vi "Recipe Label Changed-Event.vi"(8 "error in (no error)":errorcluster, 10 "New Label":string, 11 "Recipe Window in":refnum<class "Recipe Window.lvclass">) -> (0 "error out":errorcluster, 3 "Recipe Window out":refnum<class "Recipe Window.lvclass">)   [LabVIEW 2021, in "Recipe.lvlib" / "Recipe Window.lvclass"]
uses:
  Recipe Window.lvclass
  C:/Program Files (x86)/National Instruments/LabVIEW 2021/vi.lib/MGI/Monitored Actor/Monitored Actor/Monitored Actor/Monitored Actor.lvclass
  C:/Program Files (x86)/National Instruments/LabVIEW 2021/vi.lib/ActorFramework/Actor/Actor.lvclass
  <vilib>/ActorFramework/Actor/Actor.lvclass/Actor.ctl
  Main Window Interface Messages/Recipe Label Changed Msg/Recipe Label Changed Msg.lvclass/Recipe Label Changed Msg.ctl
  <vilib>/ActorFramework/Message Enqueuer/Message Enqueuer.lvclass/Message Enqueuer.ctl
  <vilib>/ActorFramework/Message Enqueuer/Enqueue.vi
  Main Window Interface Messages/Recipe Label Changed Msg/Recipe Label Changed Msg.lvclass
  C:/Program Files (x86)/National Instruments/LabVIEW 2021/vi.lib/ActorFramework/Message/Message.lvclass
  <vilib>/ActorFramework/Message Priority Queue/Priority Enqueue.vi
  <vilib>/MGI/Monitored Actor/Monitored Actor/Monitored Actor/Monitored Actor.lvclass
  <vilib>/ActorFramework/Actor/Actor.lvclass
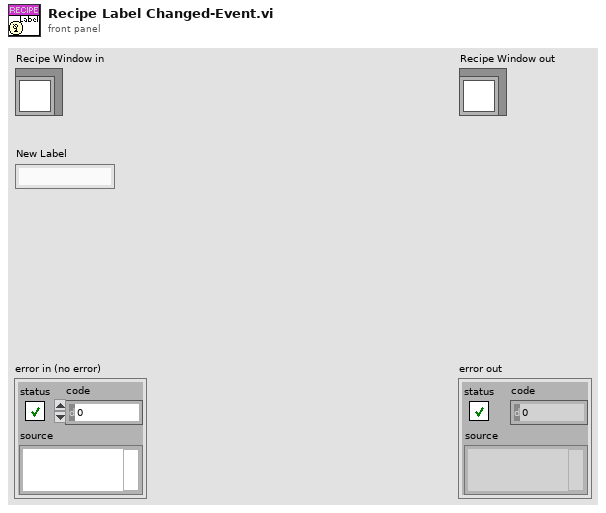
[diagram p1: front panel]
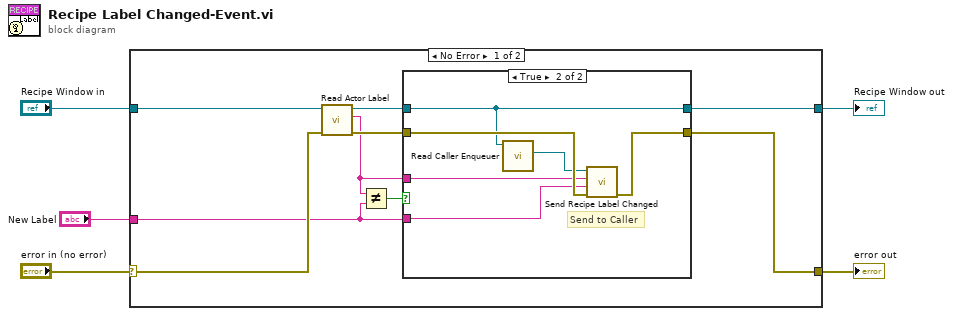
[diagram p0: block diagram]
diagram:
  n1 = case shown="No Error" "error in (no error)" {
    selector: "error in (no error)" -> [w9 w24]
    tunnel: [w14 w24] -> w3
    tunnel: [w13 w23] -> w2
    tunnel: "Recipe Window in" -> [w12 w23]
    tunnel: "New Label" -> [w7 _]
    frame No Error {
      n2 = call <vilib>:"Read Actor Label.vi"("error in (no error)"=w9, "Monitored Actor in"=w12) -> ("error out"=w10:errorcluster, "Actor Label"=w6:string, "Monitored Actor out"=w11:refnum<class "Recipe Window.lvclass">)  [unwired: 7 in]
      n3 = Not Equal?(x=w6, y=w7) -> (x != y?=w8:bool)
      n4 = case shown="True" w8 {
        tunnel: [w15 w17] -> w14
        tunnel: [w16 w21] -> w13
        tunnel: w11 -> [w16 w21]
        tunnel: w10 -> [w15 w22]
        tunnel: w7 -> [_ w18]
        tunnel: w6 -> [_ w19]
        frame False {
        }
        frame True {
          # "Send to Caller"
          n5 = call <vilib>:"Read Caller Enqueuer.vi"("Actor"=w21) -> ("Caller Enqueuer"=w20:refnum<class "Message Enqueuer.lvclass">)  [unwired: 10 in]
          n6 = call "Send Recipe Label Changed.vi"("error in (no error)"=w22, "New Label"=w18, "Old Label"=w19, "Message Enqueuer"=w20) -> ("error out"=w17:errorcluster)  [unwired: 6 in, 1 out]
        }
      }
    }
    frame Error {
    }
  }
  "error out" <- w3
  "Recipe Window out" <- w2
